vi "Find Build Specs.vi"(8 "error in":errorcluster, 11 "project path":path) -> (0 "error out":errorcluster, 3 "build specs":T1)   [LabVIEW 2020, in "Template Tool.lvlib"]
uses:
  Template Tool.lvlib
  Project Build Specs.ctl
  <vilib>/regexp/Match Regular Expression.xnode
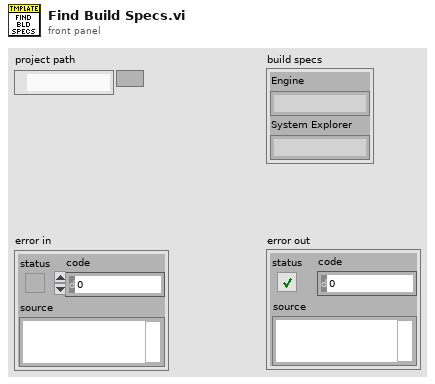
[diagram p1: front panel]
types:
  T1 = typedef "Template Tool.lvlib/Project Build Specs.ctl" = cluster{"Engine":string, "System Explorer":string}
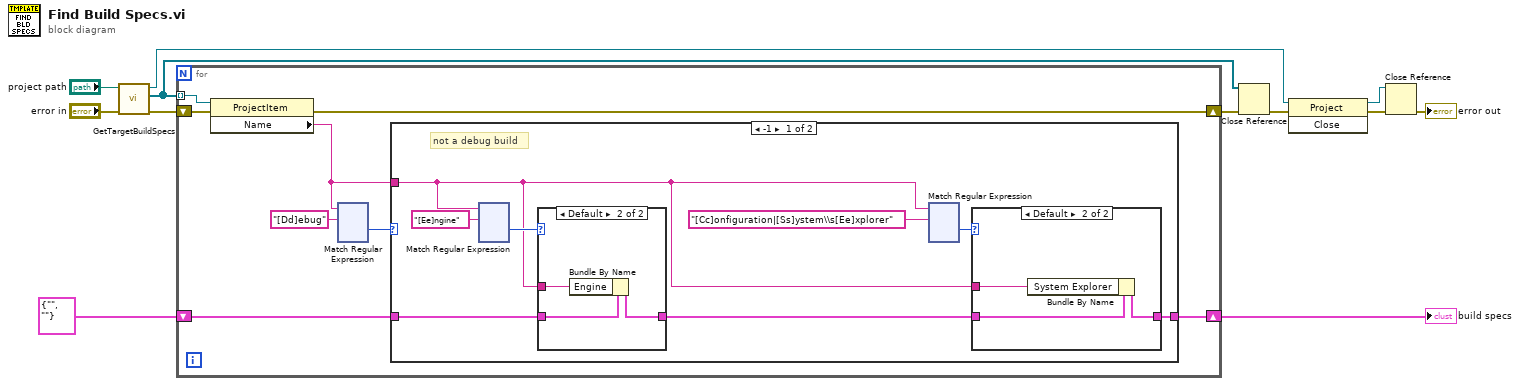
[diagram p0: block diagram]
diagram:
  n1 = call <vilib>:"GetTargetBuildSpecs.vi"("error in (no error)"="error in", "Path to project"="project path") -> ("error out"=w10:errorcluster, "buildspec refs"=w7:refnum<vi>[], "project ref"=w6:refnum<vi>)  [unwired: 7 in]
  n2 = for {
    shift-right: [w18] -> w9
    shift-left: w10 -> [w20]
    tunnel: w7 -> [w19] mode=indexing
    shift-right: [w13] -> w2
    shift-left: T1 {"Engine"="", "System Explorer"=""} ("Project Build Specs") -> [w14]
    n3 = property class="ProjectItem"(reference=w19, error in=w20) -> (error out=w18:errorcluster, "Name"=w15:string)  [unwired: 1 out]
    n4 = xnode "Match Regular Expression"("input string"=w15, "regular expression"="[Dd]ebug") -> ("offset past match"=w16:i32)  [unwired: 4 in, 4 out]
    n5 = case shown="-1" w16 {
      tunnel: w15 -> [w22 _]
      tunnel: w14 -> [w27 w265]
      tunnel: [w21 w265] -> w13
      frame -1 {
        # "not a debug build"
        n6 = xnode "Match Regular Expression"("input string"=w22, "regular expression"="[Ee]ngine") -> ("offset past match"=w26:i32)  [unwired: 4 in, 4 out]
        n7 = case shown="Default" w26 {
          tunnel: w27 -> [w147 w150]
          tunnel: [w147 w149] -> w23
          tunnel: w22 -> [_ w148]
          frame -1 {
          }
          frame Default {
            n8 = Bundle By Name(cluster=w150, "Engine"=w148) -> (w149:T1)
          }
        }
        n9 = xnode "Match Regular Expression"("input string"=w22, "regular expression"="[Cc]onfiguration|[Ss]ystem\\s[Ee]xplorer") -> ("offset past match"=w24:i32)  [unwired: 4 in, 4 out]
        n10 = case shown="Default" w24 {
          tunnel: w23 -> [w143 w146]
          tunnel: [w143 w145] -> w21
          tunnel: w22 -> [_ w144]
          frame -1 {
          }
          frame Default {
            n11 = Bundle By Name(cluster=w146, "System Explorer"=w144) -> (w145:T1)
          }
        }
      }
      frame Default {
        # "debug build - ignore"
      }
    }
  }
  "build specs" <- w2
  n12 = Close Reference(reference=w7, error in (no error)=w9) -> (error out=w8:errorcluster)
  n13 = invoke class="Project" method="Close"(reference=w6, error in=w8) -> (reference out=w4:refnum<vi>, error out=w5:errorcluster)  [unwired: 1 in, 1 out]
  n14 = Close Reference(reference=w4, error in (no error)=w5) -> (error out=→"error out":errorcluster)
